vi "Omron Serial FINS-Release.vi"(8 "error in":errorcluster, 11 "Buffer Data":T1={"VISA Resource Name"="", "Wait For Read(ms)"=50, "Command Code"=enum."Memory area read", "Command String"="", "Read Bytes"=0, "Response String"=""}) -> (0 "error out":errorcluster)   [LabVIEW 2016]
uses:
  Data Def/Omron Serial FINS-Buffer Data.ctl
  Data Def/Omron Serial FINS-Command Code.ctl
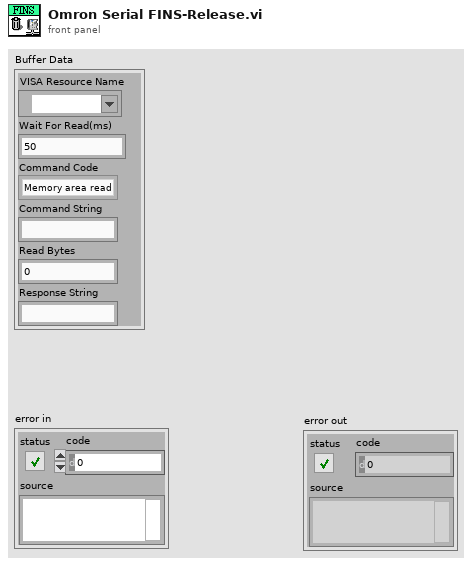
[diagram p1: front panel]
types:
  T1 = typedef "Omron Serial FINS-Buffer Data.ctl" = cluster{"VISA Resource Name":refnum<visa-resource-name>, "Wait For Read(ms)":u32, "Command Code":T2, "Command String":string, "Read Bytes":u32, "Response String":string}
  T2 = typedef "Omron Serial FINS-Command Code.ctl" = enum16{"Memory area read", "Memory area write"}
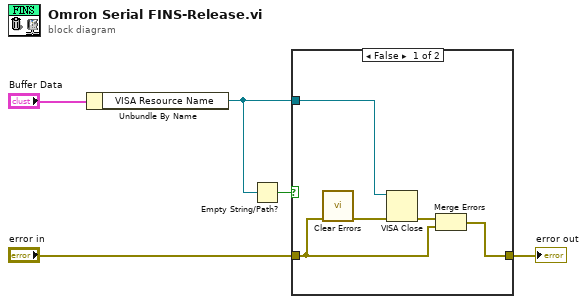
[diagram p0: block diagram]
diagram:
  n1 = Unbundle By Name("Buffer Data") -> ("VISA Resource Name"=w3:refnum<visa-resource-name>)
  n2 = Empty String/Path?(string/path=w3) -> (empty?=w5:bool)
  n3 = case shown="False" w5 {
    tunnel: "error in" -> [w6 w11]
    tunnel: w3 -> [w9 _]
    tunnel: [w7 w11] -> w2
    frame False {
      n4 = call <vilib>:"Clear Errors.vi"("error in (no error)"=w6) -> ("error out"=w10:errorcluster)  [unwired: 5 in, 1 out]
      n5 = VISA Close(VISA resource name=w9, error in (no error)=w10) -> (error out=w8:errorcluster)
      n6 = Merge Errors(w8, w6) -> (w7:errorcluster)
    }
    frame True {
    }
  }
  "error out" <- w2
